vi "Set TextAlignment.vi"(8 "error in (no error)":errorcluster, 10 "TextAlignment":i32(ring)=32 items=["TopLeft"=1, "TopCenter"=2, "TopRight"=4, "MiddleLeft"=16, "MiddleCenter"=32, "MiddleRight"=64, "BottomLeft"=256, "BottomCenter"=512, "BottomRight"=1024], 11 "View in":refnum<class "Cell View.lvclass">) -> (0 "error out":errorcluster, 3 "View out":refnum<class "Cell View.lvclass">)   [LabVIEW 2024, in "Cell View.lvclass"]
uses:
  Cell View.lvclass
  Cell View.lvclass/Cell View.ctl
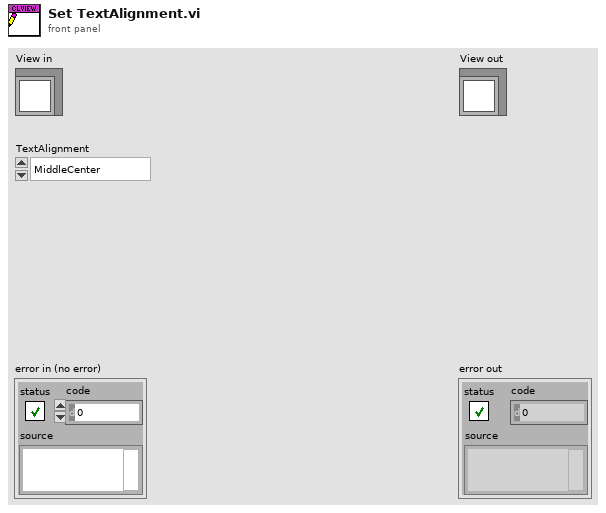
[diagram p1: front panel]
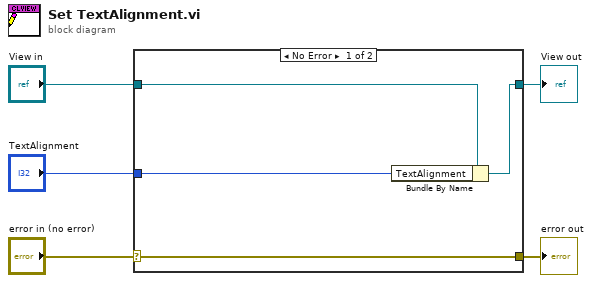
[diagram p0: block diagram]
diagram:
  n1 = case shown="No Error" "error in (no error)" {
    selector: "error in (no error)" -> [w9 w10]
    tunnel: [w9 w10] -> w4
    tunnel: [w7 w11] -> w2
    tunnel: "View in" -> [w8 w11]
    tunnel: "TextAlignment" -> [w6 _]
    frame No Error {
      n2 = Bundle By Name(cluster=w8, "TextAlignment"=w6) -> (w7:refnum<class "Cell View.lvclass">)
    }
    frame Error {
    }
  }
  "error out" <- w4
  "View out" <- w2
